vi "Application_unloadViIfExisting.vi"(0 "VIName":string, 1 "VI Refnum":refnum<vi>, 5 "error in (no error)":errorcluster, 9 "UnregisterInTable":bool) -> (14 "VIName (dup)":string, 15 "Unloaded":bool, 19 "error out":errorcluster)   [LabVIEW 2016]
doc: "Schliesst eine VI Referenz falls diese im Memory sein sollte. VI Name mit oder ohne \".vi\"\nOptional kann auch die VI Referenz verwendet werden.\n\n17.04.14 / sige"
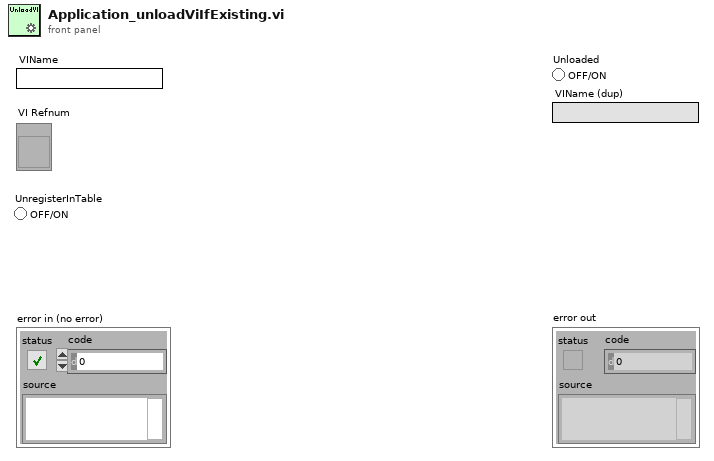
[diagram p1: front panel]
types:
  T1 = enum16{"register", "unregister", "getList", "clearList"}
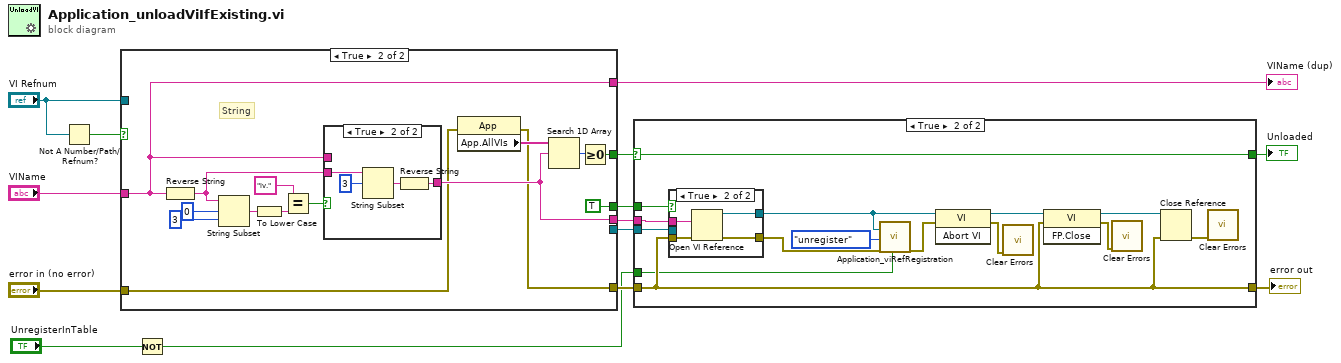
[diagram p0: block diagram]
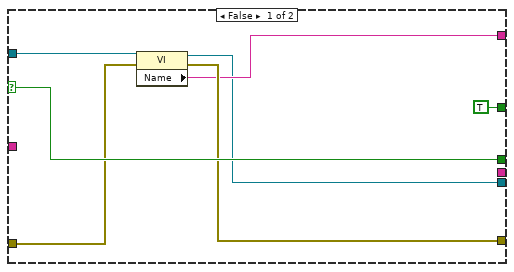
[diagram p2: hidden frame]
diagram:
  n1 = Not A Number/Path/Refnum?(number/path/refnum="VI Refnum") -> (NaN/Path/Refnum?=w10:bool)
  n2 = case shown="True" w10 {
    selector: w10 -> [w21 _]
    tunnel: [TRUE w34] -> w14
    tunnel: "VIName" -> [_ w25]
    tunnel: [_ w27] -> w11
    tunnel: "VI Refnum" -> [w19 _]
    tunnel: [w16 w25] -> w7
    tunnel: [w21 TRUE] -> w6
    tunnel: "error in (no error)" -> [w18 w23]
    tunnel: [w17 w22] -> w3
    tunnel: [w15 _] -> w4
    frame False {
      n3 = property class="VI"(reference=w19, error in=w18) -> (reference out=w15:refnum<vi>, error out=w17:errorcluster, "Name"=w16:string)
    }
    frame True {
      # "String"
      n4 = Reverse String(1:w25) -> (0:w26:string)
      n5 = String Subset(string=w26, offset (0)=0, length (rest)=3 ("length (rest)")) -> (substring=w31:string)
      n6 = To Lower Case(string=w31) -> (all lower case string=w30:string)
      n7 = Equal?(x="iv.", y=w30) -> (x = y?=w28:bool)
      n8 = case shown="True" w28 {
        tunnel: w25 -> [w37 _]
        tunnel: [w37 w39] -> w27
        tunnel: w26 -> [_ w40]
        frame False {
        }
        frame True {
          n9 = String Subset(string=w40, offset (0)=3) -> (substring=w41:string)  [unwired: 1 in]
          n10 = Reverse String(1:w41) -> (0:w39:string)
        }
      }
      n11 = property class="App"(error in=w23) -> (error out=w22:errorcluster, "App.AllVIs"=w36:string[])  [unwired: 1 in, 1 out]
      n12 = Search 1D Array(1D array=w36, element=w27) -> (index of element=w35:i32)  [unwired: 1 in]
      n13 = Greater Or Equal To 0?(x=w35) -> (x >= 0?=w34:bool)
    }
  }
  "VIName (dup)" <- w7
  n14 = Not(x="UnregisterInTable") -> (.not. x?=w1:bool)
  n15 = case shown="True" w14 {
    selector: w14 -> [w42 w56]
    tunnel: w11 -> [_ w58]
    tunnel: [w42 w56] -> w13
    tunnel: w3 -> [w43 w52]
    tunnel: [w43 w52] -> w12
    tunnel: w6 -> [_ w50]
    tunnel: w4 -> [_ w49]
    tunnel: w1 -> [_ w45]
    frame False {
    }
    frame True {
      n16 = case shown="True" w50 {
        tunnel: w58 -> [_ w64]
        tunnel: [w60 w63] -> w46
        tunnel: [w59 w62] -> w47
        tunnel: w52 -> [w59 w61]
        tunnel: w49 -> [w60 _]
        frame False {
        }
        frame True {
          n17 = Open VI Reference(vi path=w64, error in (no error)=w61) -> (vi reference=w63:refnum<vi>, error out=w62:errorcluster)  [unwired: 4 in]
        }
      }
      n18 = call "Application_viRefRegistration.vi"("VI Refnum"=w46, "Command"=T1."unregister", "error in (no error)"=w47, "Skip"=w45) -> ("error out"=w48:errorcluster)  [unwired: 14 in, 1 out]
      n19 = invoke class="VI" method="Abort VI"(reference=w46, error in=w48) -> (reference out=w53:refnum<vi>, error out=w51:errorcluster)  [unwired: 1 in, 1 out]
      n20 = call <vilib>:"Clear Errors.vi"("error in (no error)"=w51) -> ()  [unwired: 5 in, 2 out]
      n21 = invoke class="VI" method="FP.Close"(reference=w53, error in=w52) -> (reference out=w55:refnum<vi>, error out=w54:errorcluster)  [unwired: 1 in, 1 out]
      n22 = call <vilib>:"Clear Errors.vi"("error in (no error)"=w54) -> ()  [unwired: 5 in, 2 out]
      n23 = Close Reference(reference=w55, error in (no error)=w52) -> (error out=w57:errorcluster)
      n24 = call <vilib>:"Clear Errors.vi"("error in (no error)"=w57) -> ()  [unwired: 5 in, 2 out]
    }
  }
  "Unloaded" <- w13
  "error out" <- w12
